vi "AuMT8852B Path Offset Mode.vi"(5 "Mode (Off)":enum16{"Off", "Fixed", "Table"}(ring), 7 "Set/Get (Set)":enum16{"Set", "Get"}(ring), 8 "error in (no error)":errorcluster, 10 "Script (3)":i32=3, 11 "VISA session":refnum<visa-resource-name>) -> (0 "error out":errorcluster, 2 "error code":i32, 3 "VISA session out":refnum<visa-resource-name>, 4 "Mode out":enum16{"Off", "Fixed", "Table"}(ring))   [LabVIEW 2017]
doc: "Anritsu MT8852B Bluetooth Tester\n\nSpecifies how path loss will be applied to the transmitter power.\n\nINPUTS\nSet/Get - whether the path offset mode is being written or read.\nScript - test script for which the path offset applies.\nMode - whether no path offset, a fixed offset, or an offset table will be applied.\n\nOUTPUTS\nMode out - type of offset currently being applied."
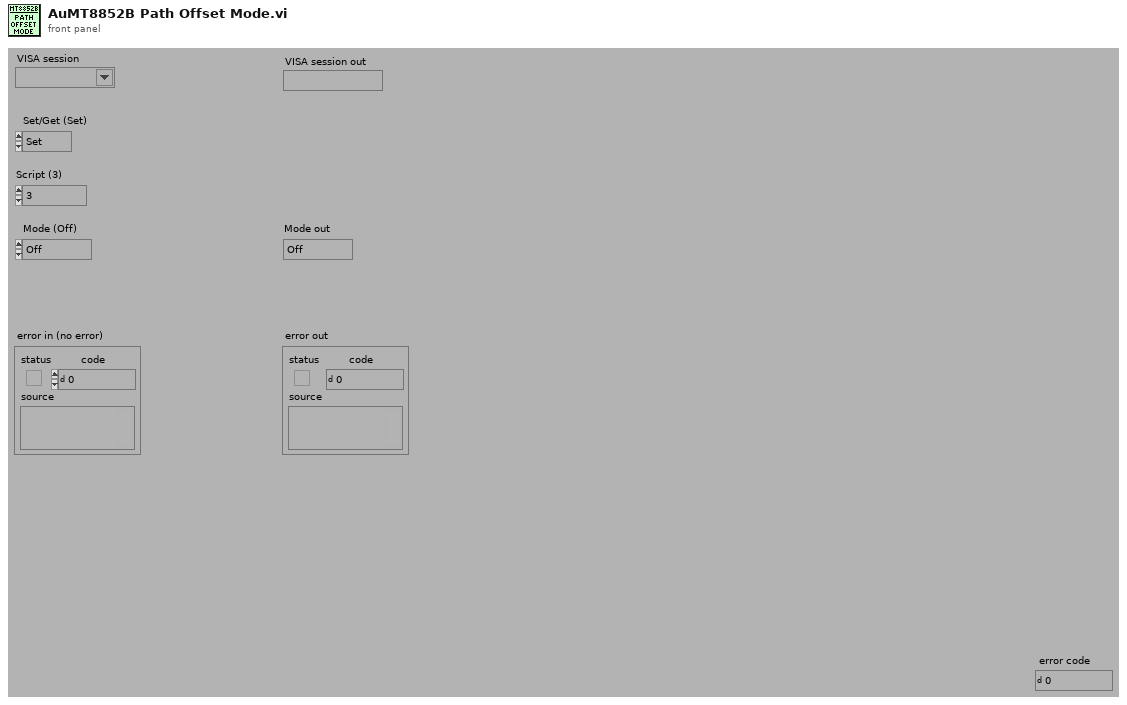
[diagram p1: front panel]
types:
  T1 = enum16{"Simulate", "Range check", "Cache", "Query instrument status"}
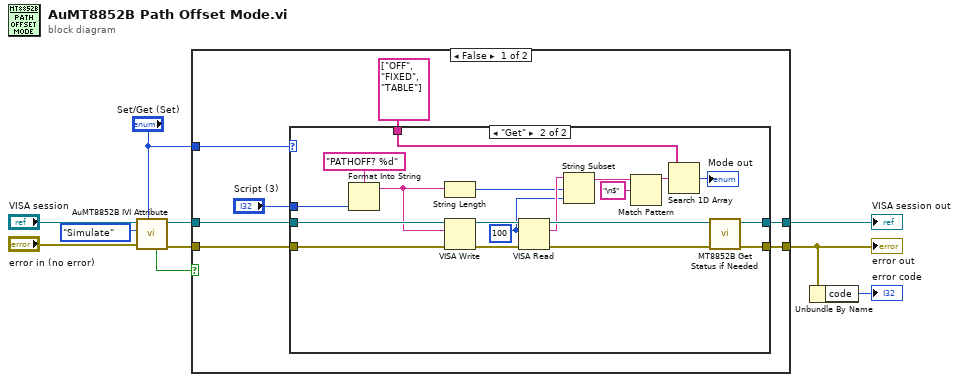
[diagram p0: block diagram]
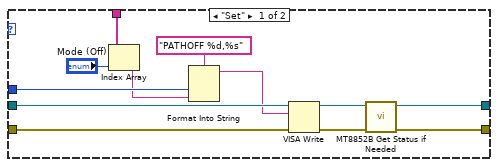
[diagram p2: hidden frame]
diagram:
  n1 = call <instrlib>:"AuMT8852B IVI Attribute.vi"("Set/Get (Set)"="Set/Get (Set)", "error in (no error)"="error in (no error)", "Flag (Simulate)"=T1."Simulate", "VISA session"="VISA session") -> ("error out"=w5:errorcluster, "VISA session out"=w7:refnum<visa-resource-name>, "Value out"=w4:bool)  [unwired: 5 in]
  n2 = case shown="False" w4 {
    tunnel: [w17 w50] -> w1
    tunnel: [w16 w49] -> w10
    tunnel: w7 -> [w15 w49]
    tunnel: w5 -> [w14 w50]
    tunnel: "Set/Get (Set)" -> [w13 _]
    frame False {
      n3 = case shown="\"Get\"" w13 {
        tunnel: [w29 w48] -> w17
        tunnel: [w28 w47] -> w16
        tunnel: w15 -> [w25 w46]
        tunnel: w14 -> [w24 w45]
        tunnel: "Script (3)" -> [w22 w43]
        tunnel: string[] ["OFF", "FIXED", "TABLE"] ("Array Constant") -> [w19 w32]
        frame "Set" {
          n4 = Index Array(array=w19, index="Mode (Off)") -> (element=w20:string)
          n5 = Format Into String(format string="PATHOFF %d,%s" ("Format String"), w22, w20) -> (resulting string=w21:string)  [unwired: 2 in, 1 out]
          n6 = VISA Write(VISA resource name=w25, write buffer=w21, error in (no error)=w24) -> (VISA resource name out=w27:refnum<visa-resource-name>, error out=w26:errorcluster)  [unwired: 1 out]
          n7 = call <instrlib>:"MT8852B Get Status if Needed.vi"("error in (no error)"=w26, "VISA session"=w27) -> ("error out"=w29:errorcluster, "VISA session out"=w28:refnum<visa-resource-name>)  [unwired: 8 in]
        }
        frame "Get" {
          w30 = u32 100 ("byte count (0)")
          n8 = Format Into String(format string="PATHOFF? %d" ("Format String"), w43) -> (resulting string=w34:string)  [unwired: 2 in, 1 out]
          n9 = String Length(string=w34) -> (length=w33:i32)
          n10 = VISA Write(VISA resource name=w46, write buffer=w34, error in (no error)=w45) -> (VISA resource name out=w42:refnum<visa-resource-name>, error out=w41:errorcluster)  [unwired: 1 out]
          n11 = VISA Read(VISA resource name=w42, byte count=w30, error in (no error)=w41) -> (VISA resource name out=w40:refnum<visa-resource-name>, read buffer=w35:string, error out=w39:errorcluster)  [unwired: 1 out]
          n12 = String Subset(string=w35, offset (0)=w33, length (rest)=w30) -> (substring=w37:string)
          n13 = Match Pattern(string=w37, regular expression="\n$") -> (before substring=w36:string)  [unwired: 1 in, 3 out]
          n14 = Search 1D Array(1D array=w32, element=w36) -> (index of element=→"Mode out":i32)  [unwired: 1 in]
          n15 = call <instrlib>:"MT8852B Get Status if Needed.vi"("error in (no error)"=w39, "VISA session"=w40) -> ("error out"=w48:errorcluster, "VISA session out"=w47:refnum<visa-resource-name>)  [unwired: 8 in]
        }
      }
    }
    frame True {
    }
  }
  "error out" <- w1
  "VISA session out" <- w10
  n16 = Unbundle By Name(w1) -> ("code"=→"error code":i32)
